vi "Pump Read Data.vi"(8 "error in (no error)":errorcluster, 11 "VISA Refnum in":refnum<visa-resource-name>) -> (0 "error out":errorcluster, 2 "Variant":variant)   [LabVIEW 2020, in "Pump.lvlib"]
uses:
  Pump.lvlib
  <instrlib>/WM Pump/WM Pump.lvlib
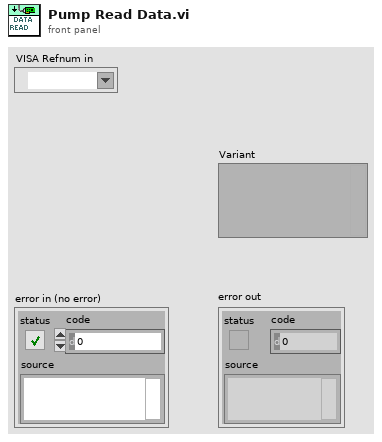
[diagram p1: front panel]
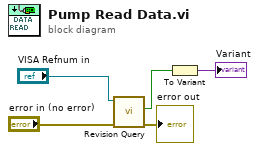
[diagram p0: block diagram]
diagram:
  n1 = call <instrlib>:"Revision Query.vi"("error in (no error)"="error in (no error)", "VISA resource name"="VISA Refnum in") -> ("error out"=→"error out":errorcluster, "Started"=w1:bool)  [unwired: 7 in, 1 out]
  n2 = To Variant(anything=w1) -> (Variant=→"Variant":variant)
